vi "Read File.vi"(8 "error in (no error)":errorcluster, 11 "Setup File in":refnum<class "Setup File.lvclass">) -> (0 "error out":errorcluster, 1 "CHANNELS":i32[](array[numeric]), 2 "Array":string[][](array[string]), 3 "Setup File out":refnum<class "Setup File.lvclass">)   [LabVIEW 2018, in "Setup File.lvclass"]
uses:
  Setup File.lvclass
  Setup File.lvclass/Setup File.ctl
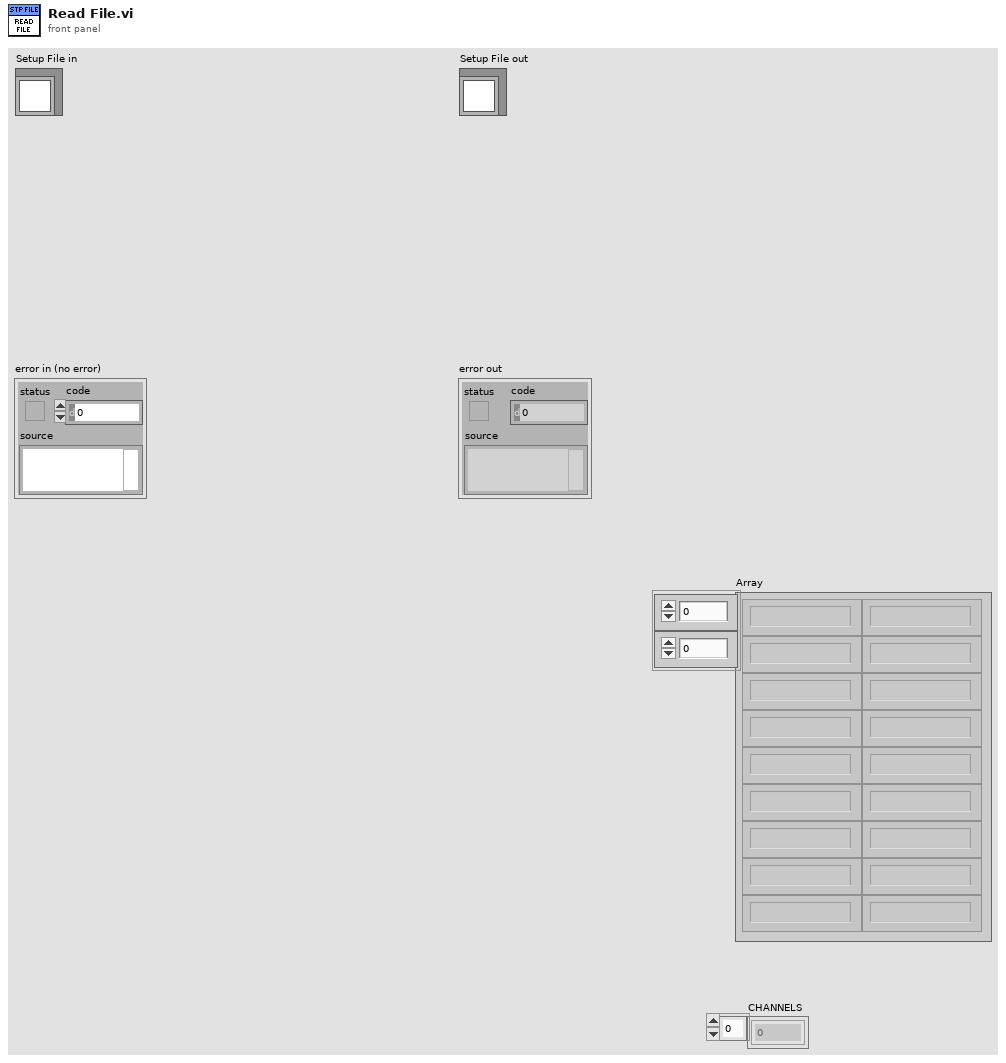
[diagram p1: front panel]
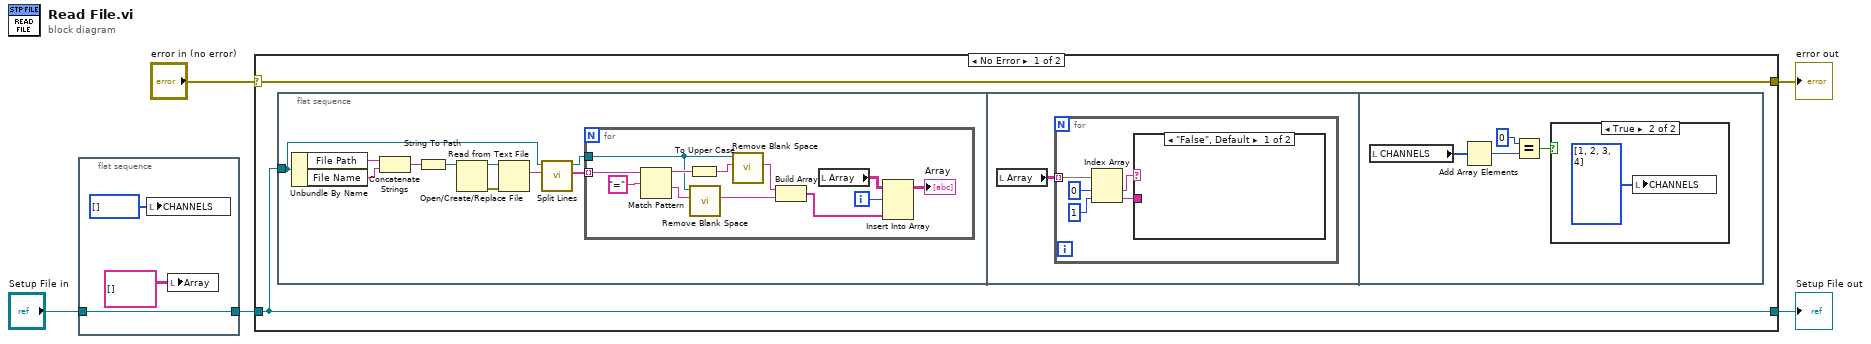
[diagram p0: block diagram]
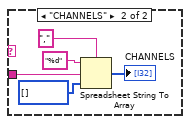
[diagram p2: hidden frame]
diagram:
  n1 = flat-sequence {
    tunnel: "Setup File in" -> [w7]
    tunnel: [w7] -> w1
    frame #0 {
      n2 = local write "CHANNELS"(i32[] []) -> ()
      n3 = local write "Array"(string[][] [] ("Array")) -> ()
    }
  }
  n4 = case shown="No Error" "error in (no error)" {
    selector: "error in (no error)" -> [w10 w49]
    tunnel: [w10 w49] -> w4
    tunnel: [w9 w50] -> w3
    tunnel: w1 -> [w9 w50]
    frame No Error {
      n5 = flat-sequence {
        tunnel: w9 -> [w11]
        frame #0 {
          n6 = Unbundle By Name(w11) -> ("File Path"=w15:string, "File Name"=w14:string)
          n7 = Concatenate Strings(w15, w14) -> (w16:string)
          n8 = String To Path(string=w16) -> (path=w17:path)
          n9 = Open/Create/Replace File(file path (use dialog)=w17) -> (refnum out=w13:refnum<file>, error out=w12:errorcluster)  [unwired: 5 in, 1 out]
          n10 = Read from Text File(file (use dialog)=w13, error in=w12) -> (text=w19:string)  [unwired: 2 in, 3 out]
          n11 = call "Split Lines.vi"("spreadsheet string"=w19, "Setup File in"=w11) -> ("array"=w18:string[], "Setup File out"=w20:refnum<class "Setup File.lvclass">)  [unwired: 7 in, 1 out]
          n12 = for {
            tunnel: w18 -> [w32] mode=indexing
            tunnel: w20 -> [w29]
            i -> [w22]
            n13 = Match Pattern(string=w32, regular expression="=" ("search string/char (-)")) -> (before substring=w30:string, after substring=w28:string)  [unwired: 1 in, 2 out]
            n14 = To Upper Case(1:w30) -> (0:w27:string)
            n15 = call "Remove Blank Space.vi"("string in"=w28, "Setup File in"=w29) -> ("string out"=w26:string)  [unwired: 7 in, 2 out]
            n16 = call "Remove Blank Space.vi"("string in"=w27, "Setup File in"=w29) -> ("string out"=w25:string)  [unwired: 7 in, 2 out]
            n17 = Build Array(w25, w26) -> (w24:string[])
            n18 = local read "Array"() -> (w23:string[][])
            n19 = Insert Into Array(array=w23, index (row)=w22, new element=w24) -> (→"Array":string[][])  [unwired: 1 in]
          }
        }
        frame #1 {
          n20 = local read "Array"() -> (w33:string[][])
          n21 = for {
            tunnel: w33 -> [w36] mode=indexing
            n22 = Index Array(array=w36, index #1=0 ("index"), index #2=1 ("index")) -> (element #1=w35:string, element #2=w34:string)
            n23 = case shown="\"False\", Default" w35 {
              tunnel: w34 -> [_ w39]
              frame "False", Default {
              }
              frame "CHANNELS" {
                n24 = Spreadsheet String To Array(delimiter (Tab)="," ("format string"), format string="%d", spreadsheet string=w39, array type (2D Dbl)=i32[] []) -> (array=→"CHANNELS":i32[])
              }
            }
          }
        }
        frame #2 {
          n25 = local read "CHANNELS"() -> (w47:i32[])
          n26 = Add Array Elements(numeric array=w47) -> (sum=w46:i32)
          n27 = Equal?(x=0, y=w46) -> (x = y?=w45:bool)
          n28 = case shown="True" w45 {
            frame False {
            }
            frame True {
              n29 = local write "CHANNELS"(i32[] [1, 2, 3, 4]) -> ()
            }
          }
        }
      }
    }
    frame Error {
    }
  }
  "error out" <- w4
  "Setup File out" <- w3
